vi "ProcessEvtQDC.vi"(8 "error in":errorcluster, 9 "Encoded Data":u32[](array[numeric]), 10 "# data points in evt":i32) -> (0 "error out":errorcluster, 1 "Decoded Data":T1[](array[typedef]), 2 "# Events":u32, 3 "Overflow?":bool)   [LabVIEW 2014]
uses:
  QDCDataCluster.ctl
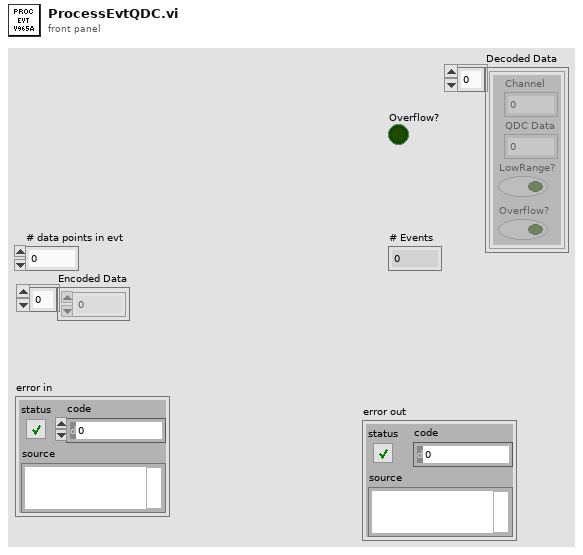
[diagram p1: front panel]
types:
  T1 = typedef "QDCDataCluster.ctl" = cluster{"Channel":u8, "QDC Data":sgl, "LowRange?":bool, "Overflow?":bool}
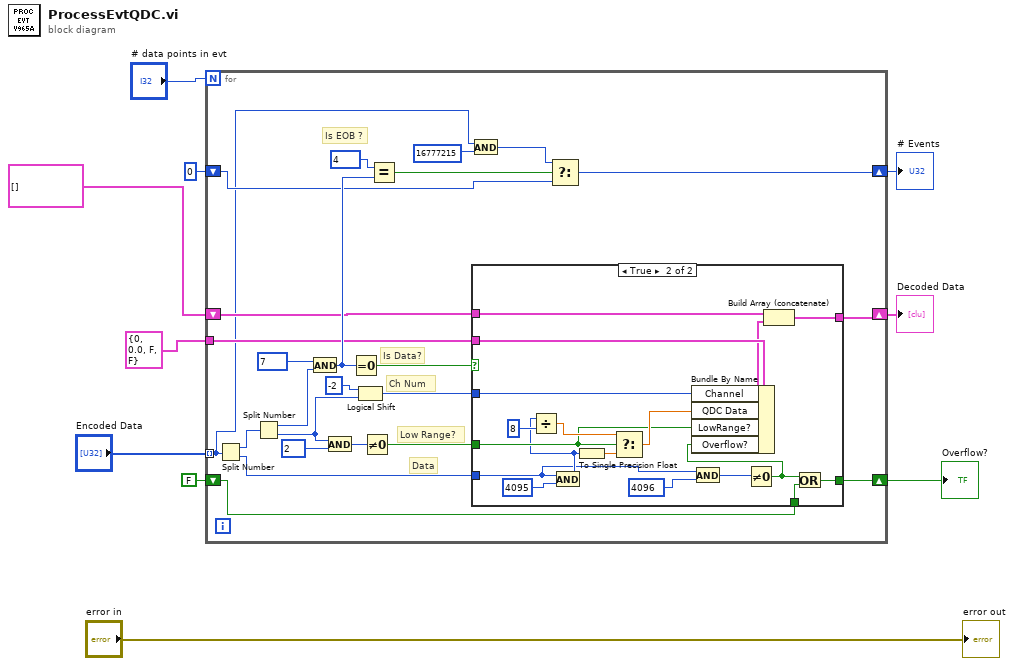
[diagram p0: block diagram]
diagram:
  n1 = for {
    N: "# data points in evt" -> [_]
    tunnel: "Encoded Data" -> [w13] mode=indexing
    tunnel: T1 {"Channel"=0, "QDC Data"=0.0, "LowRange?"=FALSE, "Overflow?"=FALSE} -> [w21]
    shift-right: [w14] -> w1
    shift-left: T1[] [] ("appended array") -> [w20]
    shift-right: [w16] -> w6
    shift-left: u32 0 -> [w15]
    shift-right: [w12] -> w2
    shift-left: FALSE -> [w11]
    # "Is EOB ?"
    # "Data"
    # "Is Data?"
    # "Low Range?"
    # "Ch Num"
    n2 = Split Number(x=w13) -> (hi(x)=w34:u16, lo(x)=w26:u16)
    n3 = Split Number(x=w34) -> (hi(x)=w31:u8, lo(x)=w28:u8)
    n4 = And(x=u8 7, y=w31) -> (x .and. y?=w23:u8)
    n5 = And(x=w28, y=u8 2) -> (x .and. y?=w29:u8)
    n6 = Equal To 0?(x=w23) -> (x = 0?=w25:bool)
    n7 = Logical Shift(y=i16 -2, x=w28) -> (x << y=w22:u8)
    n8 = Not Equal To 0?(x=w29) -> (x != 0?=w27:bool)
    n9 = Equal?(x=u8 4, y=w23) -> (x = y?=w19:bool)
    n10 = And(x=w13, y=u32 16777215 ("x")) -> (x .and. y?=w17:u32)
    n11 = case shown="True" w25 {
      tunnel: w26 -> [_ w38]
      tunnel: w27 -> [_ w45]
      tunnel: w22 -> [_ w50]
      tunnel: w21 -> [_ w51]
      tunnel: [w36 w44] -> w14
      tunnel: w20 -> [w36 w48]
      tunnel: [w35 w40] -> w12
      tunnel: w11 -> [w35 w39]
      frame False {
      }
      frame True {
        n12 = And(x=w38, y=u16 4095) -> (x .and. y?=w42:u16)
        n13 = Divide(x=w42, y=u16 8) -> (x/y=w52:sgl)
        n14 = To Single Precision Float(number=w42) -> (single precision float=w47:sgl)
        n15 = Select(t=w52, s=w45, f=w47) -> (s? t:f=w49:sgl)
        n16 = And(x=w38, y=u16 4096) -> (x .and. y?=w41:u16)
        n17 = Not Equal To 0?(x=w41) -> (x != 0?=w37:bool)
        n18 = Bundle By Name(cluster=w51, "Channel"=w50, "QDC Data"=w49, "LowRange?"=w45, "Overflow?"=w37) -> (w46:T1)
        n19 = Build Array (concatenate)(w48, w46) -> (w44:T1[])
        n20 = Or(x=w37, y=w39) -> (x .or. y?=w40:bool)
      }
    }
    n21 = Select(t=w17, s=w19, f=w15) -> (s? t:f=w16:u32)
  }
  "# Events" <- w6
  "Overflow?" <- w2
  "Decoded Data" <- w1
  "error out" <- "error in"
